vi "Example Launcher.vi"() -> ()   [LabVIEW 2023, in "Async Methods Actor Example.lvlib"]
uses:
  Async Methods Actor Example.lvlib
  Async Methods Actor Example/Async Methods Actor Example.lvclass
  C:/Program Files/National Instruments/LabVIEW 2023/vi.lib/LS Instruments AG/Async Methods Actor/Async Methods Actor/Async Methods Actor/Async Methods Actor.lvclass
  C:/Program Files/National Instruments/LabVIEW 2023/vi.lib/ActorFramework/Actor/Actor.lvclass
  <vilib>/LS Instruments AG/Async Methods Actor/Async Methods Actor/Async Methods Actor/Running Methods Communication.ctl
  <vilib>/LS Instruments AG/Async Methods Actor/Async Methods Actor/Async Methods Actor/Async Methods Actor.lvclass/Async Methods Actor.ctl
  <vilib>/LS Instruments AG/Async Methods Actor/Async Methods Actor/Async Methods Actor/Write Running Methods Communication.vi
  <vilib>/ActorFramework/Actor/Actor.lvclass
  <vilib>/LS Instruments AG/Async Methods Actor/Async Methods Actor/Async Methods Actor/Async Methods Actor.lvclass
panel:
  out "error out":errorcluster
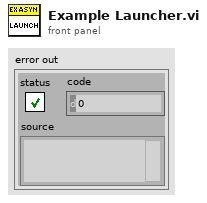
[diagram p1: front panel]
types:
  T1 = typedef "Async Methods Actor.lvlib/Async Methods Actor.lvclass/Running Methods Communication.ctl" = enum16{"None", "Notifier", "Event"}
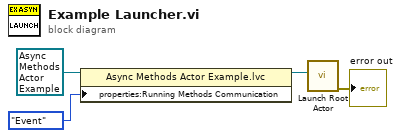
[diagram p0: block diagram]
diagram:
  n1 = property class="Async Methods Actor Example.lvc"(reference=refnum<class "Async Methods Actor Example.lvclass"> refnum ("Async Actor Example.lvlib:Async Actor Example.lvclass"), "properties:Running Methods Communication"=Running_Methods_Communication."Event" ("Running Methods Communication")) -> (reference out=w2:refnum<class "Async Methods Actor Example.lvclass">)  [unwired: 1 in, 1 out]
  n2 = call <vilib>:"Launch Root Actor.vi"("Actor"=w2) -> ("error out"=→"error out":errorcluster)  [unwired: 9 in, 1 out]
